vi "Select Channels.vi"(8 "error in (no error)":errorcluster, 10 "Channels to Highlight":string[](array[string]), 11 "Item Ref In":T1=18446744073709551615 format="%.0x") -> (0 "error out":errorcluster, 1 "Channels Selected":string[](array[string]), 3 "Dup Item Ref":T1=18446744073709551615 format="%.0x")   [LabVIEW 2012, in "Running Average Custom Device.lvlib"]
uses:
  Running Average Custom Device.lvlib
  NationalInstruments.VeriStand.SystemStorageUI
  <vilib>/NI Veristand/Custom Device API/Custom Device Item Ref.ctl
  NationalInstruments.VeriStand.SystemStorage
  <vilib>/NI Veristand/Custom Device API/Custom Device API.lvlib
panel:
  in  "Cancel":bool
  in  "Ok":bool
  in  "TreeBrowserWF":refnum<k24>(container)
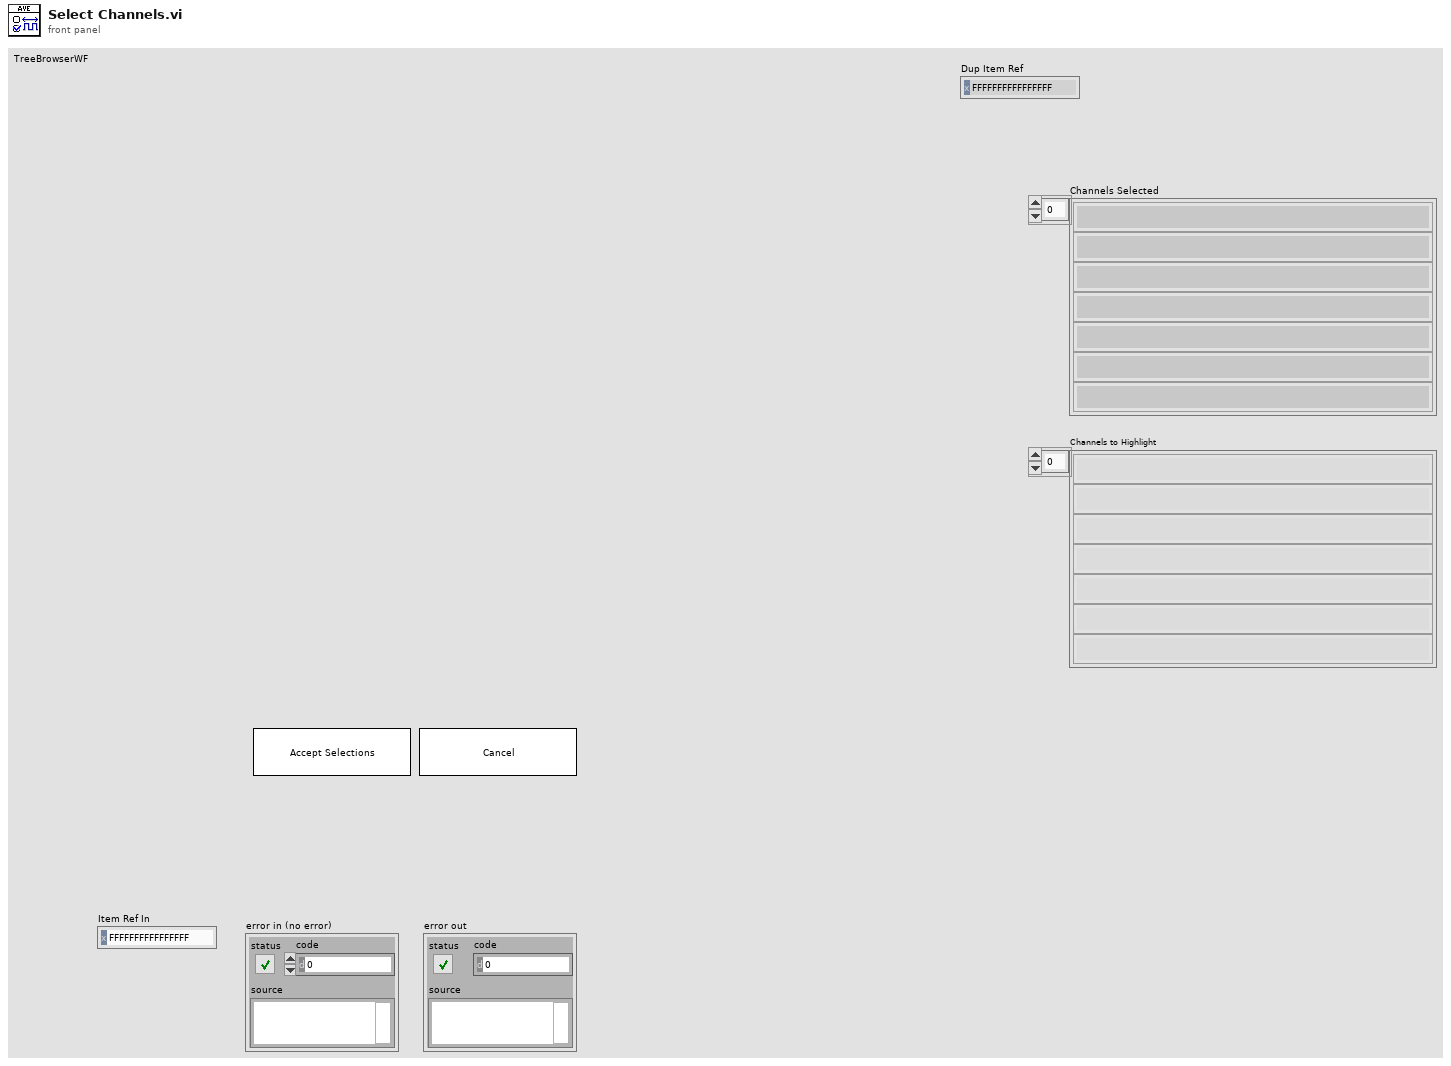
[diagram p1: front panel]
types:
  T1 = typedef "Custom Device API.lvlib/Custom Device Item Ref.ctl" = u64
  T2 = typedef "Custom Device API.lvlib/Custom Device Pointer.ctl" = refnum<k24>
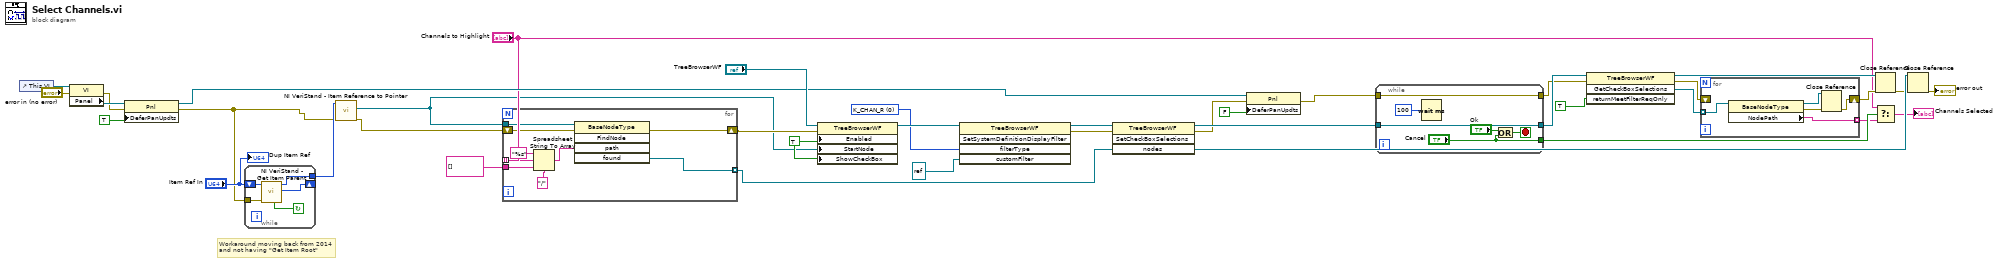
[diagram p0: block diagram]
diagram:
  w30 = u8 0 items=["K_CHAN_R", "K_CHAN_W", "K_CHAN_RW", "K_CHAN_VOLT", "K_CHAN_FAULT", "K_ALL", "K_CUSTOM", "K_CHAN_R_VIS", "K_CHAN_W_VIS", "K_CHAN_RW_VIS", "K_CHAN_VOLT_VIS", "K_CHAN_FAULT_VIS", "K_WAVE", "K_WAVE_VIS", "K_WAVE_DBL", "K_WAVE_CDB", "K_WAVE_DBL_VIS", "K_WAVE_CDB_VIS"] ("filterType")
  w38 = TRUE ("Enabled")
  # "Workaround moving back from 2014\nand not having \"Get Item Root\""
  n1 = control-ref of="This VI"() -> (w21:refnum<vi>)
  n2 = property class="VI"(reference=w21, error in="error in (no error)") -> (error out=w6:errorcluster, "Panel"=w20:refnum<vi>)  [unwired: 1 out]
  n3 = property class="Pnl"(reference=w20, error in=w6, "DeferPanUpdts"=TRUE ("Defer Panel Updates")) -> (reference out=w16:refnum<vi>, error out=w2:errorcluster)
  n4 = while {
    shift-right: [w41] -> _
    shift-left: "Item Ref In" -> [w44]
    tunnel: w2 -> [w43]
    tunnel: [w42] -> w3
    stop <- w40 continue-if-true
    n5 = call <vilib>:"NI VeriStand - Get Item Parent.vi"("error in (no error)"=w43, "Item Ref in"=w44) -> ("Parent Ref"=w41:T1, "Item Ref out"=w42:T1, "Found"=w40:bool)  [unwired: 6 in, 1 out]
  }
  n6 = call <vilib>:"NI VeriStand - Item Reference to Pointer.vi"("error in (no error)"=w2, "Item Ref in"=w3) -> ("error out"=w9:errorcluster, "Node Pointer"=w1:T2)  [unwired: 6 in, 2 out]
  n7 = for {
    tunnel: w1 -> [w53]
    tunnel: "Channels to Highlight" -> [w52] mode=indexing
    tunnel: string[] [] -> [w51]
    tunnel: [w48] -> w12 mode=indexing
    shift-right: [w45] -> w11
    shift-left: w9 -> [w46]
    n8 = Spreadsheet String To Array(delimiter (Tab)="/", format string="%s", spreadsheet string=w52, array type (2D Dbl)=w51) -> (array=w49:string[])
    n9 = invoke class="BaseNodeType" method="FindNode"(reference=w53, error in=w46, "path"=w49) -> (error out=w45:errorcluster, "found"=w48:refnum<k24>)  [unwired: 2 in, 3 out]
  }
  n10 = property class="TreeBrowserWF"(reference="TreeBrowserWF", error in=w11, "Enabled"=w38, "StartNode"=w1, "ShowCheckBox"=w38) -> (reference out=w31:refnum<k24>)  [unwired: 1 out]
  n11 = invoke class="TreeBrowserWF" method="SetSystemDefinitionDisplayFilter"(reference=w31, "filterType"=w30, "customFilter"=refnum<k24> refnum) -> (reference out=w28:refnum<k24>, error out=w27:errorcluster)  [unwired: 2 in, 3 out]
  n12 = invoke class="TreeBrowserWF" method="SetCheckBoxSelections"(reference=w28, error in=w27, "nodes"=w12) -> (reference out=w26:refnum<k24>, error out=w18:errorcluster, "nodes"=w25:refnum<k24>[])  [unwired: 1 in, 1 out]
  n13 = property class="Pnl"(reference=w16, error in=w18, "DeferPanUpdts"=FALSE ("Defer Panel Updates")) -> (error out=w17:errorcluster)  [unwired: 1 out]
  n14 = while {
    tunnel: [w58] -> w34
    tunnel: w26 -> [w58]
    tunnel: ["Cancel"] -> w24
    tunnel: w17 -> [w54]
    tunnel: [w54] -> w8
    stop <- w56 stop-if-true
    n15 = Wait (ms)(milliseconds to wait=u32 100) -> ()  [unwired: 1 out]
    n16 = Or(x="Ok", y="Cancel") -> (x .or. y?=w56:bool)
  }
  n17 = invoke class="TreeBrowserWF" method="GetCheckBoxSelections"(reference=w34, error in=w8, "returnMeetFilterReqOnly"=TRUE) -> (reference out=w35:refnum<k24>, error out=w33:errorcluster, "GetCheckBoxSelections"=w37:refnum<k24>[])  [unwired: 1 in, 1 out]
  n18 = for {
    tunnel: w37 -> [w64] mode=indexing
    tunnel: [w63] -> w23 mode=indexing
    shift-right: [w60] -> w32
    shift-left: w33 -> [_]
    n19 = property class="BaseNodeType"(reference=w64) -> (reference out=w62:refnum<k24>, error out=w61:errorcluster, "NodePath"=w63:string)  [unwired: 1 in]
    n20 = Close Reference(reference=w62, error in (no error)=w61) -> (error out=w60:errorcluster)
  }
  n21 = Close Reference(reference=w35, error in (no error)=w32) -> (error out=w10:errorcluster)
  n22 = Select(t="Channels to Highlight", s=w24, f=w23) -> (s? t:f=→"Channels Selected":string[])
  n23 = Close Reference(reference=w25, error in (no error)=w10) -> (error out=→"error out":errorcluster)
  "Dup Item Ref" <- "Item Ref In"
